vi "Is Diamond.vi"(0 "ROI Descriptor (Diamond Match)":T1={"Global Rectangle"=[530, 711, 555, 739], "Contours"=[{"ID"=enum."External", "Type"=12, "Coordinates"=[530, 711, 555, 739, 0]}]} {"Contours"."Type" items=["No Selection", "Point", "Line", "Rectangle", "Oval", "Polygon", "Freehand Region", "Annulus", "Unused2", "Unused3", "Broken Line", "Freehand Line", "Rotated Rectangle"]}, 3 "error in":errorcluster) -> (10 "error out":errorcluster)   [LabVIEW 2015]
uses:
  <vilib>/vision/NI_Vision_Development_Module.lvlib
panel:
  in  "SS File Path":path
  out "Image Out":T2(plugin-control)
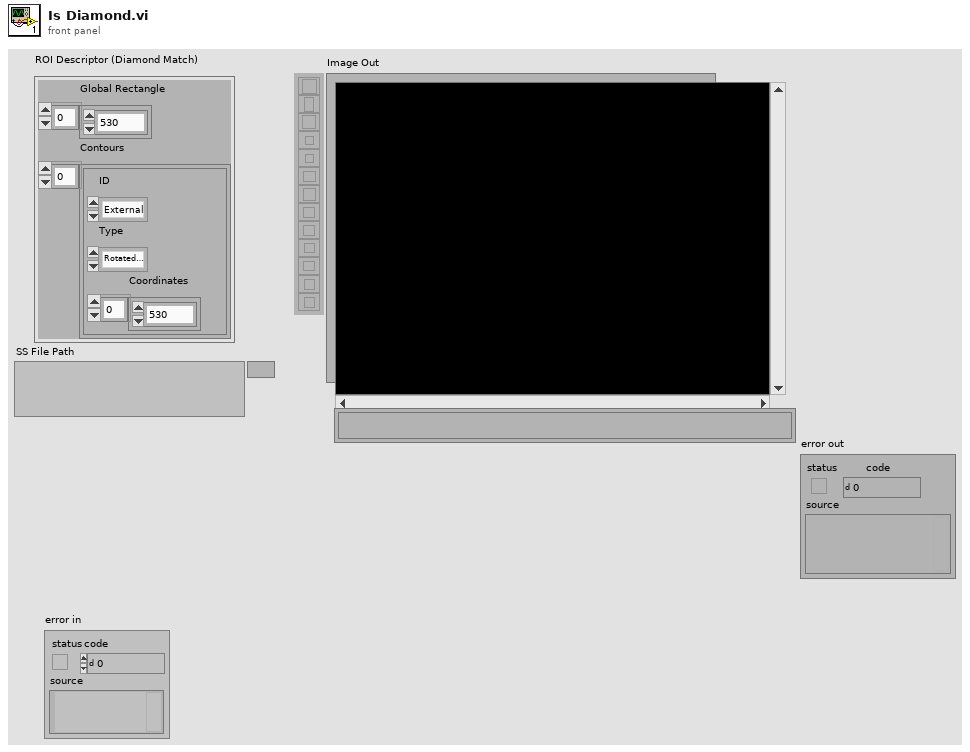
[diagram p1: front panel]
types:
  T1 = cluster{"Global Rectangle":i32[], "Contours":cluster{"ID":enum32{"External", "Internal"}, "Type":u32, "Coordinates":i32[]}[]}
  T2 = typedef "IMAQ Image.ctl" = refnum<image>
  T3 = cluster{"Number of Matches Requested":i32, "Minimum Match Score":sgl, "Angle Ranges":cluster{"Start Angle":sgl, "End Angle":sgl}[]}
  T4 = typedef "Image Type" = u32
  T5 = cluster{"Position":cluster{"x":sgl, "y":sgl}, "Angle":sgl, "Scale":sgl, "Score":sgl, "Bounding Box":cluster{"x":sgl, "y":sgl}[]}[]
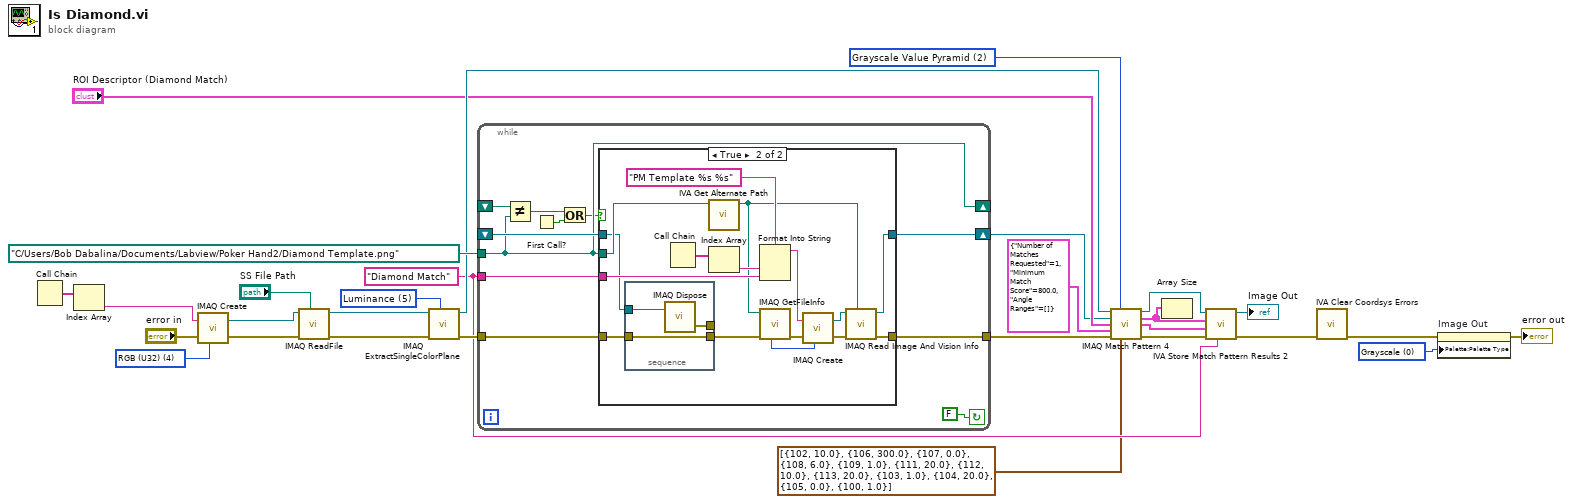
[diagram p0: block diagram]
diagram:
  w2 = u32 0 items=["Grayscale", "Binary", "Gradient", "Rainbow", "Temperature", "User Defined", "Binary 16 Bit", "Gradient 16 Bit", "Rainbow 16 Bit", "Temperature 16 Bit", "User Defined 16 Bit"] ("Palette Type")
  w15 = 2 items=["All", "Low Discrepancy Sampling", "Grayscale Value Pyramid", "Gradients Pyramid"] ("Algorithm")
  w12 = "Diamond Match" ("Step Name")
  w22 = 5 items=["Red", "Green", "Blue", "Hue", "Saturation", "Luminance", "Value", "Intensity"] ("Color Plane")
  w23 = T4 4 items=["Grayscale (U8)", "Grayscale (I16)", "Grayscale (SGL)", "Complex (CSG)", "RGB (U32)", "HSL (U32)", "RGB (U64)", "Grayscale (U16)"] ("Image Type")
  n1 = Call Chain() -> (call chain=w25:string[])
  n2 = Index Array(array=w25) -> (element=w24:string)  [unwired: 1 in]
  n3 = call "IMAQ Create"("Image Name"=w24, "Image Type"=w23, "error in (no error)"="error in") -> ("New Image"=w28:T2, "error out"=w27:errorcluster)  [unwired: 1 in, 1 out]
  n4 = call "IMAQ ReadFile"("File Path"="SS File Path", "error in (no error)"=w27, "Image"=w28) -> ("error out"=w29:errorcluster, "Image Out"=w21:T2)  [unwired: 2 in, 5 out]
  n5 = call "IMAQ ExtractSingleColorPlane"("Color Plane"=w22, "error in (no error)"=w29, "Image Src"=w21) -> ("error out"=w20:errorcluster, "Image Dst Out"=w18:T2)  [unwired: 1 in, 6 out]
  n6 = while {
    shift-right: [w40] -> w9
    shift-left: _ -> [w39]
    tunnel: [w37] -> w8
    tunnel: w20 -> [w36]
    tunnel: path "C:/Users/Bob Dabalina/Documents/Labview/Poker Hand2/Diamond Template.png" ("Template File Path") -> [w33]
    tunnel: w12 -> [w35]
    shift-right: [w33] -> _
    shift-left: _ -> [w34]
    stop <- FALSE continue-if-true
    n7 = Not Equal?(x=w34, y=w33) -> (x != y?=w31:bool)
    n8 = First Call?() -> (First Call?: T/F=w32:bool)
    n9 = Or(x=w31, y=w32) -> (x .or. y?=w30:bool)
    n10 = case shown="True" w30 {
      tunnel: [w42 w56] -> w40
      tunnel: w39 -> [w42 w48]
      tunnel: [w41 w53] -> w37
      tunnel: w36 -> [w41 w47]
      tunnel: w33 -> [_ w49]
      tunnel: w35 -> [_ w50]
      frame False {
      }
      frame True {
        n11 = stacked-sequence {
          tunnel: w48 -> [w61]
          tunnel: w47 -> [w60]
          tunnel: [w60] -> w43
          tunnel: [w59] -> _
          frame #0 {
            n12 = call "IMAQ Dispose"("Image"=w61) -> ("error out"=w59:errorcluster)  [unwired: 2 in, 3 out]
          }
        }
        n13 = Call Chain() -> (call chain=w52:string[])
        n14 = call <vilib>:"IVA Get Alternate Path.vi"("Path In"=w49) -> ("Path Out"=w45:path)  [unwired: 10 out]
        n15 = Index Array(array=w52) -> (element=w51:string)  [unwired: 1 in]
        n16 = Format Into String(format string="PM Template %s %s" ("Image Name"), w51, w50) -> (resulting string=w58:string)  [unwired: 2 in, 1 out]
        n17 = call "IMAQ GetFileInfo"("error in (no error)"=w43, "File Path"=w45) -> ("error out"=w44:errorcluster, "Image Type"=w46:T4)  [unwired: 3 in, 5 out]
        n18 = call "IMAQ Create"("Image Name"=w58, "Image Type"=w46, "error in (no error)"=w44) -> ("New Image"=w55:T2, "error out"=w54:errorcluster)  [unwired: 1 in, 1 out]
        n19 = call "IMAQ Read Image And Vision Info"("File Path"=w45, "error in (no error)"=w54, "Image"=w55) -> ("error out"=w53:errorcluster, "Image Out"=w56:T2)  [unwired: 1 in, 6 out]
      }
    }
  }
  n20 = call "IMAQ Match Pattern 4"("Image"=w18, "Algorithm"=w15, "Template Image"=w9, "ROI Descriptor"="ROI Descriptor (Diamond Match)", "Parameters"=T3 {"Number of Matches Requested"=1, "Minimum Match Score"=800.0, "Angle Ranges"=[]}, "error in (no error)"=w8, "Advanced Options"=cluster{"Item":u16, "Value":dbl}[] [{"Item"=102, "Value"=10.0}, {"Item"=106, "Value"=300.0}, {"Item"=107, "Value"=0.0}, {"Item"=108, "Value"=6.0}, {"Item"=109, "Value"=1.0}, {"Item"=111, "Value"=20.0}, {"Item"=112, "Value"=10.0}, {"Item"=113, "Value"=20.0}, {"Item"=103, "Value"=1.0}, {"Item"=104, "Value"=20.0}, {"Item"=105, "Value"=0.0}, {"Item"=100, "Value"=1.0}]) -> ("Image (duplicate)"=w16:T2, "Matches (pixel)"=w11:T5, "Matches (real-world)"=w10:T5, "error out"=w17:errorcluster)  [unwired: 4 in, 1 out]
  n21 = Array Size(array=w11) -> ()  [unwired: 1 out]
  n22 = call <vilib>:"IVA Store Match Pattern Results 2.vi"("Step Name"=w12, "error in (no error)"=w17, "Matches (real-world)"=w10, "Matches (pixel)"=w11, "Image in"=w16) -> ("error out"=w7:errorcluster, "Image dup"=→"Image Out":T2)  [unwired: 1 in, 4 out]
  n23 = call <vilib>:"IVA Clear Coordsys Errors.vi"("error in (no error)"=w7) -> ("error out"=w6:errorcluster)  [unwired: 10 in]
  n24 = property on="Image Out" class="ImageControl"(error in=w6, "Palette:Palette Type"=w2) -> (error out=→"error out":errorcluster)  [unwired: 1 in, 1 out]
